vi "Remove Item.vi"(8 "error in (no error)":errorcluster, 11 "Listbox Refs in":T1 {"Section Ref" format="%.0x"}) -> (0 "error out":errorcluster, 3 "Listbox Refs out":T1 {"Section Ref" format="%.0x"})   [LabVIEW 2016, in "FPGA Addon System Explorer.lvlib"]
uses:
  FPGA Addon System Explorer.lvlib
  Listbox Cluster.ctl
  <vilib>/NI Veristand/Custom Device API/Custom Device Item Ref.ctl
  Shared/Constants.vi
  <vilib>/NI VeriStand/Custom Device API/Custom Device API.lvlib
  Shared/FPGA Addon Shared.lvlib
  VeriStand-FPGA-Resource-Manager/Source/FPGA Resource Manager System Definition.lvlib
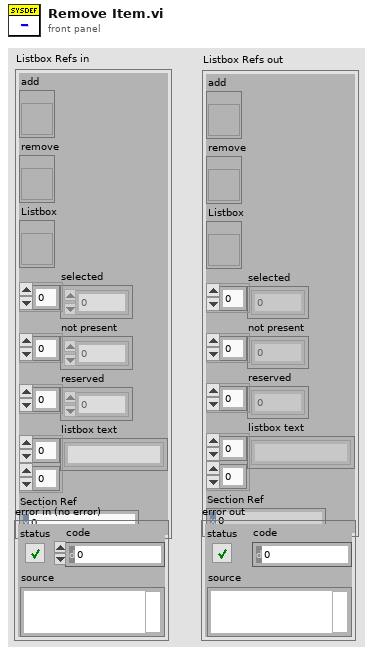
[diagram p1: front panel]
types:
  T1 = typedef "FPGA Addon System Explorer.lvlib/Listbox Cluster.ctl" = cluster{"add":refnum<vi>, "remove":refnum<vi>, "Listbox":refnum<vi>, "selected":i32[], "not present":i32[], "reserved":i32[], "listbox text":string[][], "Section Ref":T2}
  T2 = typedef "Custom Device API.lvlib/Custom Device Item Ref.ctl" = u64
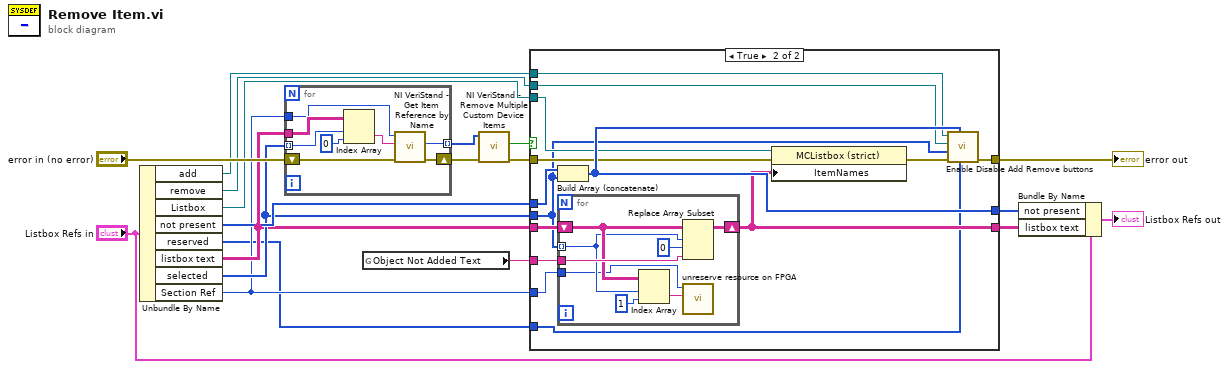
[diagram p0: block diagram]
diagram:
  n1 = Unbundle By Name("Listbox Refs in") -> ("add"=w5:refnum<vi>, "remove"=w4:refnum<vi>, "Listbox"=w3:refnum<vi>, "not present"=w15:i32[], "reserved"=w1:i32[], "listbox text"=w6:string[][], "selected"=w7:i32[], "Section Ref"=w2:T2)
  n2 = for {
    tunnel: w7 -> [w21] mode=indexing
    tunnel: w6 -> [w27]
    tunnel: w2 -> [w23]
    tunnel: [w24] -> w11 mode=indexing
    shift-right: [w20] -> w12
    shift-left: "error in (no error)" -> [w25]
    n3 = Index Array(array=w27, index (row)=w21, index (col)=0 ("disabled index (col)")) -> (element=w22:string)
    n4 = call <vilib>:"NI VeriStand - Get Item Reference by Name.vi"("error in (no error)"=w25, "Item Name"=w22, "Parent Ref in"=w23) -> ("error out"=w20:errorcluster, "Item Ref"=w24:T2)  [unwired: 5 in, 2 out]
  }
  n5 = global read "Constants.vi" "Object Not Added Text"() -> (w8:string)
  n6 = call <vilib>:"NI VeriStand - Remove Multiple Custom Device Items.vi"("error in (no error)"=w12, "Item Refs in"=w11) -> ("error out"=w10:errorcluster, "Deleted?"=w9:bool)  [unwired: 8 in]
  n7 = case shown="True" w9 {
    tunnel: [w29 w44] -> w13
    tunnel: w10 -> [w29 w39]
    tunnel: w7 -> [_ w33]
    tunnel: w6 -> [w30 w43]
    tunnel: w8 -> [_ w42]
    tunnel: [w30 w34] -> w18
    tunnel: w15 -> [w28 w41]
    tunnel: [w28 w40] -> w17
    tunnel: w5 -> [_ w37]
    tunnel: w4 -> [_ w36]
    tunnel: w3 -> [_ w35]
    tunnel: w2 -> [_ w32]
    tunnel: w1 -> [_ w31]
    frame False {
    }
    frame True {
      n8 = Build Array (concatenate)(w41, w33) -> (w40:i32[])
      n9 = for {
        tunnel: w33 -> [w48] mode=indexing
        shift-right: [w52] -> w34
        shift-left: w43 -> [w49]
        tunnel: w42 -> [w50]
        tunnel: w32 -> [w46]
        n10 = Index Array(array=w49, index (row)=w48, index (col)=1 ("disabled index (col)")) -> (element=w45:string)
        n11 = Replace Array Subset(array=w49, new element=w50, index (row)=w48, index (col)=0 ("disabled index (col)")) -> (w52:string[][])
        n12 = call "unreserve resource on FPGA.vi"("Name in bitfile"=w45, "Item Ref in"=w46) -> ()  [unwired: 7 in, 3 out]
      }
      n13 = property class="MCListbox (strict)"(reference=w35, error in=w39, "ItemNames"=w34) -> (error out=w38:errorcluster)  [unwired: 1 out]
      n14 = call "Enable Disable Add Remove buttons.vi"("reserved item indexes"=w31, "not present item indexes"=w40, "error in (no error)"=w38, "selected items"=w33, "remove button"=w36, "add button"=w37) -> ("error out"=w44:errorcluster)  [unwired: 5 in]
    }
  }
  "error out" <- w13
  n15 = Bundle By Name(cluster="Listbox Refs in", "not present"=w17, "listbox text"=w18) -> (→"Listbox Refs out":T1)
